vi "setIDN.vi"(4 "Version":string, 6 "Serial Number":string, 8 "error in (no error)":errorcluster, 9 "Name":string, 10 "Vendor":string, 11 "Instrument in":refnum<class "Instrument.lvclass">) -> (0 "error out":errorcluster, 3 "Instrument out":refnum<class "Instrument.lvclass">)   [LabVIEW 2019, in "Instrument.lvlib" / "Instrument.lvclass"]
uses:
  Instrument.lvclass
  Typedefs/Instrument.IDN--cluster.ctl
  Typedefs/Instrument.ProtectedCommands--Enum.ctl
  API/Instrument.sendMessageToProcess (variant).vi
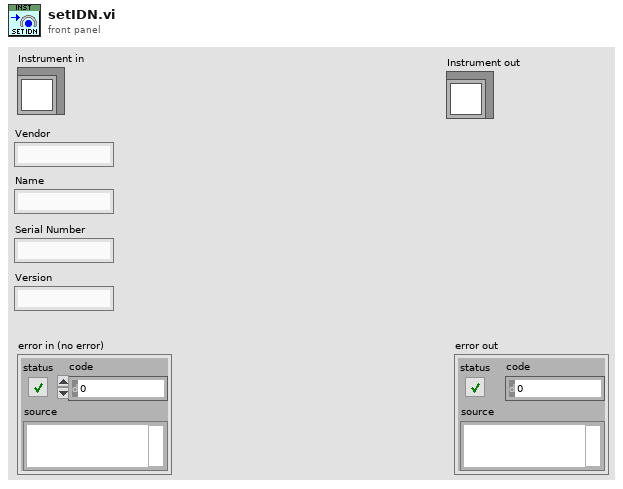
[diagram p1: front panel]
types:
  T1 = typedef "Instrument.lvlib/Instrument.lvclass/Instrument.ProtectedCommands--Enum.ctl" = enum16{"setConfiguration", "setIDN", "setAll", "setAllData"}
  T2 = typedef "Instrument.lvlib/Instrument.lvclass/Instrument.IDN--cluster.ctl" = cluster{"vendor":string, "model":string, "serial":string, "firmware":string}
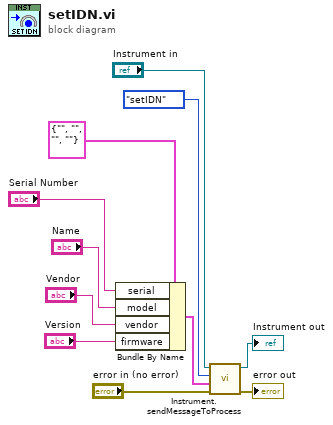
[diagram p0: block diagram]
diagram:
  n1 = Bundle By Name(cluster=T2 {"vendor"="", "model"="", "serial"="", "firmware"=""} ("IDN"), "serial"="Serial Number", "model"="Name", "vendor"="Vendor", "firmware"="Version") -> (w3:T2)
  n2 = call-poly "Instrument.sendMessageToProcess.vi"("error in (no error)"="error in (no error)", "Data"=w3, "Command"=Instrument.ProtectedCommands--Enum."setIDN" ("PrivateCommands"), "Instrument"="Instrument in") -> ("error out"=→"error out":errorcluster, "Instrument out"=→"Instrument out":refnum<class "Instrument.lvclass">)  [unwired: 6 in]
